vi "comparsion_funcion.vi"() -> ()   [LabVIEW 2019]
panel:
  out "x <= y?":bool
  out "x >= y?":bool
  out "x < y?":bool
  out "x > y?":bool
  out "x != y?":bool
  out "x = y?":bool
  in  "x":dbl
  in  "y":dbl
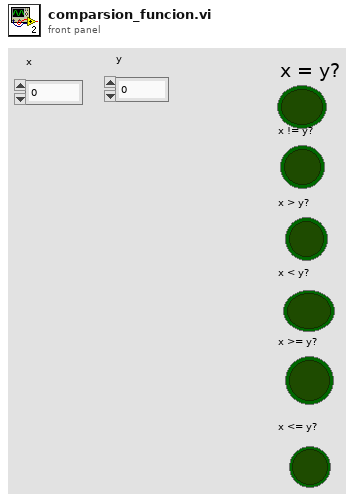
[diagram p1: front panel]
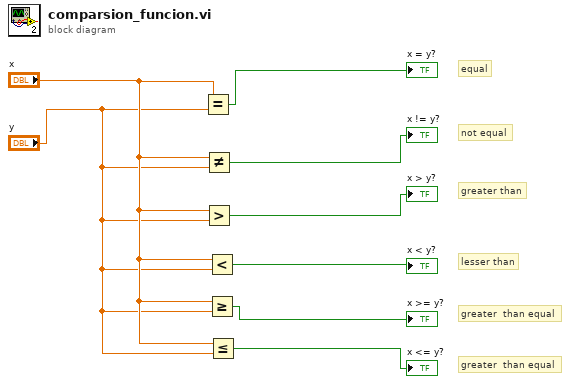
[diagram p0: block diagram]
diagram:
  # "greater  than equal"
  # "greater  than equal"
  # "lesser than"
  # "not equal"
  # "greater than"
  # "equal"
  n1 = Equal?(x="x", y="y") -> (x = y?=→"x = y?":bool)
  n2 = Not Equal?(x="x", y="y") -> (x != y?=→"x != y?":bool)
  n3 = Greater?(x="x", y="y") -> (0:→"x > y?":bool)
  n4 = Less?(x="x", y="y") -> (x < y?=→"x < y?":bool)
  n5 = Greater Or Equal?(x="x", y="y") -> (x >= y?=→"x >= y?":bool)
  n6 = Less Or Equal?(x="x", y="y") -> (x <= y?=→"x <= y?":bool)
